vi "Lift PID Control.vi"(0 "Motor DevRefs IN":T15, 5 "Operator Gamepad":T4, 7 "Lift Potentionmeter":T1, 9 "Lift Deadband":dbl, 11 "Gains":cluster{"P":dbl, "I":dbl, "D":dbl}, 12 "Time to Wait":i32, 13 "Limit":dbl) -> (4 "Motor DevRefs OUT":T15, 10 "Tolerable?":bool)   [LabVIEW 2014]
uses:
  <vilib>/Rock Robotics/WPI/MotorControl/WPI_MotorControlDeviceRef.ctl
  <vilib>/Rock Robotics/WPI/MotorControl/WPI_MotorControlType.ctl
  <vilib>/Rock Robotics/SystemInterfaces/Typedef/FPGA_TypedefDigitalModule.ctl
  <vilib>/Rock Robotics/SystemInterfaces/DIO/FPGA_DIOPWMChannel.ctl
  <vilib>/Rock Robotics/WPI/PWM/WPI_PWMDeadband.ctl
  <vilib>/Rock Robotics/WPI/CAN/Jaguar/SubVIs/WPI_CANJaguar_ControlMode.ctl
  <vilib>/Rock Robotics/WPI/CAN/TalonSRX/WPI_CANTalonSRX_APIControlMode.ctl
  <vilib>/Rock Robotics/WPI/PWM/WPI_PWMTransform_ConPane.ctl
  <vilib>/Rock Robotics/WPI/Joystick/WPI_JoystickDevRef.ctl
  <vilib>/Rock Robotics/WPI/Joystick/WPI_JoystickDeviceEnum.ctl
  <vilib>/Rock Robotics/WPI/Potentiometer/WPI_PotentiometerDevRef.ctl
  <vilib>/Rock Robotics/SystemInterfaces/Typedef/FPGA_TypedefAnalogModule.ctl
  <vilib>/Rock Robotics/SystemInterfaces/AI/FPGA_AIChannel.ctl
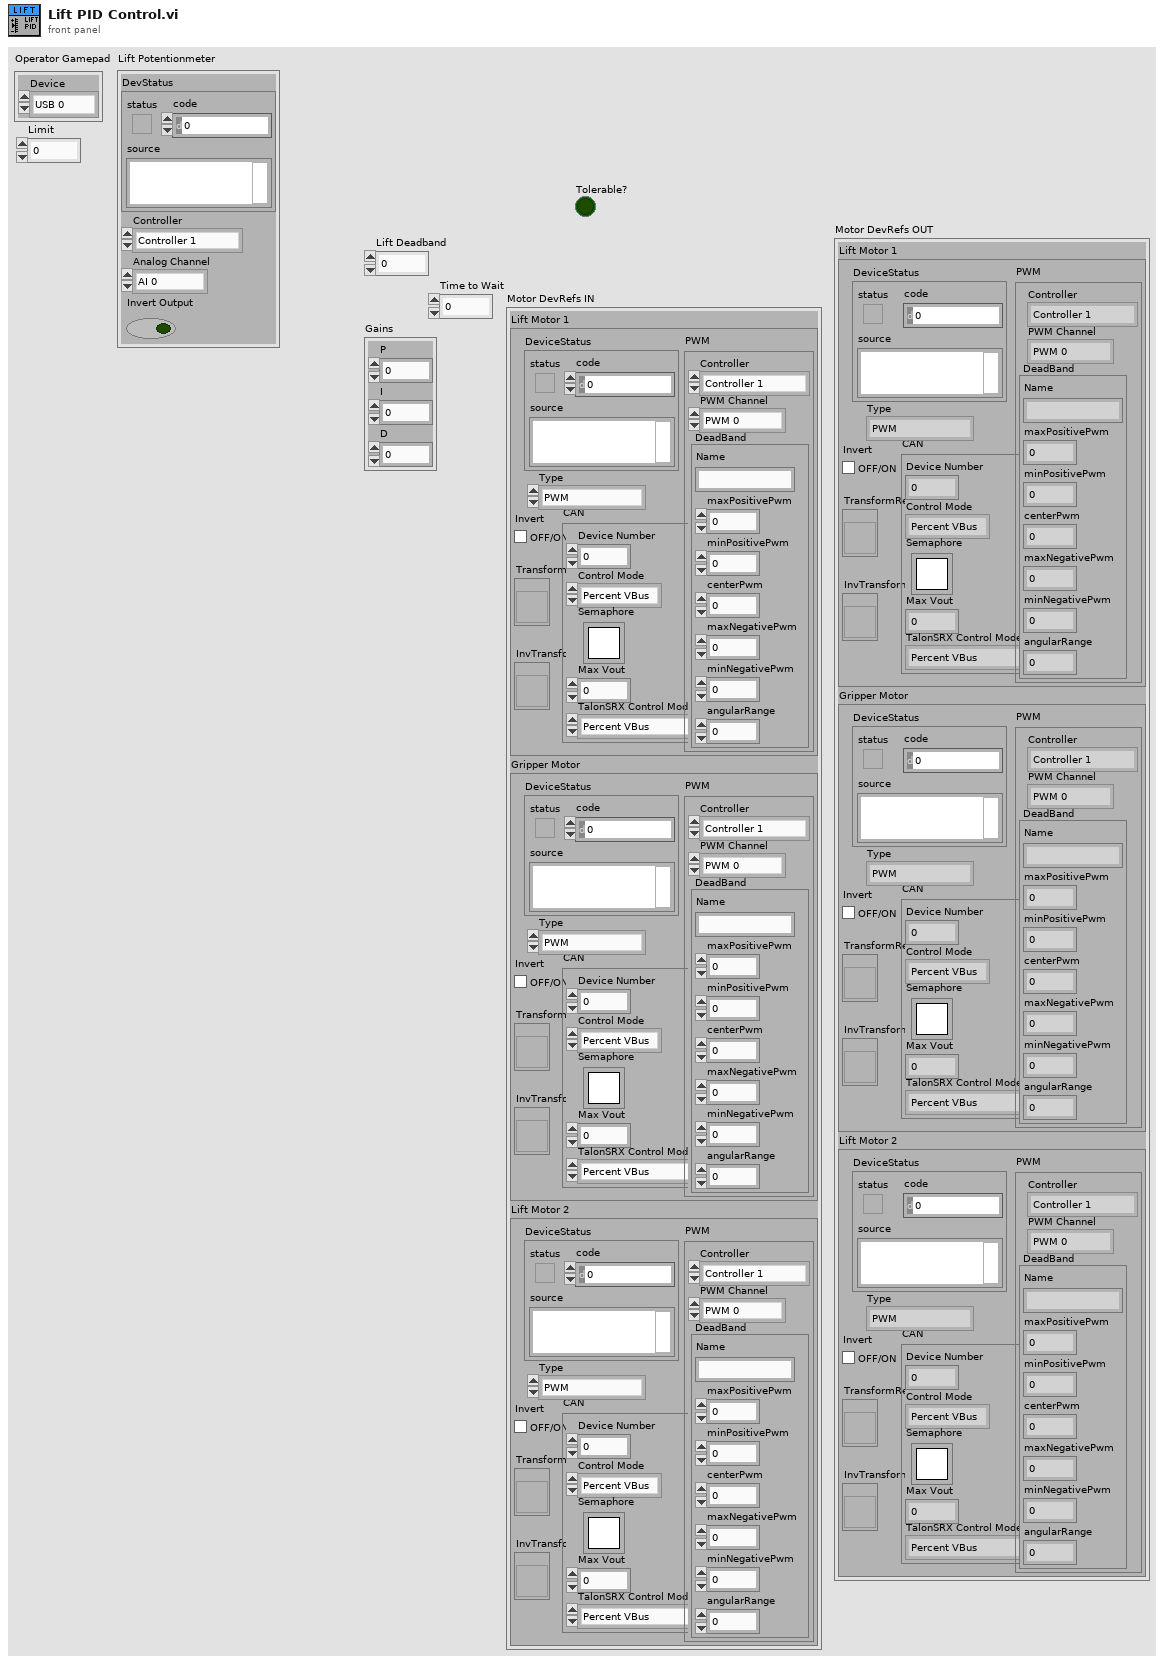
[diagram p1: front panel]
types:
  T1 = typedef "WPI_PotentiometerDevRef.ctl" = cluster{"DevStatus":errorcluster, "Controller":T2, "Analog Channel":T3, "Invert Output":bool}
  T2 = typedef "FPGA_TypedefAnalogModule.ctl" = enum16{"Controller 1"}
  T3 = typedef "FPGA_AIChannel.ctl" = enum8{"AI 0", "AI 1", "AI 2", "AI 3", "AI MXP 0", "AI MXP 1", "AI MXP 2", "AI MXP 3", "Invalid"}
  T4 = typedef "WPI_JoystickDevRef.ctl" = cluster{"Device":T5}
  T5 = typedef "WPI_JoystickDeviceEnum.ctl" = enum16{"USB 0", "USB 1", "USB 2", "USB 3", "USB 4", "USB 5"}
  T6 = typedef "WPI_MotorControlDeviceRef.ctl" = cluster{"DeviceStatus":errorcluster, "Type":T7, "PWM":cluster{"Controller":T8, "PWM Channel":T9, "DeadBand":T10}, "CAN":cluster{"Device Number":u8, "Control Mode":T11, "Semaphore":T12, "Max Vout":dbl, "TalonSRX Control Mode":T13}, "Invert":bool, "TransformRef":T14, "InvTransformRef":T14}
  T7 = typedef "WPI_MotorControlType.ctl" = enum16{"PWM", "CAN", "CANTalonSRX"}
  T8 = typedef "FPGA_TypedefDigitalModule.ctl" = enum16{"Controller 1"}
  T9 = typedef "FPGA_DIOPWMChannel.ctl" = enum8{"PWM 0", "PWM 1", "PWM 2", "PWM 3", "PWM 4", "PWM 5", "PWM 6", "PWM 7", "PWM 8", "PWM 9", "PWM MXP 0", "PWM MXP 1", "PWM MXP 2", "PWM MXP 3", "PWM MXP 4", "PWM MXP 5", "PWM MXP 6", "PWM MXP 7", "PWM MXP 8", "PWM MXP 9", "Invalid"}
  T10 = typedef "WPI_PWMDeadband.ctl" = cluster{"Name":string, "maxPositivePwm":i32, "minPositivePwm":i32, "centerPwm":i32, "maxNegativePwm":i32, "minNegativePwm":i32, "angularRange":u16}
  T11 = typedef "WPI_CANJaguar_ControlMode.ctl" = enum8{"Percent VBus", "Current", "Speed", "Position", "Voltage"}
  T12 = typedef "Semaphore RefNum" = refnum<k1>
  T13 = typedef "WPI_CANTalonSRX_APIControlMode.ctl" = enum8{"Percent VBus", "Speed", "Position", "Slave", "Unchanged / Invalid"}
  T14 = typedef "WPI_PWMTransform_ConPane.ctl" = refnum<vi>
  T15 = cluster{"Lift Motor 1":T6, "Gripper Motor":T6, "Lift Motor 2":T6}
  T16 = cluster{"Error":dbl, "millisecond timer value":u32, "To Shift Register":dbl}
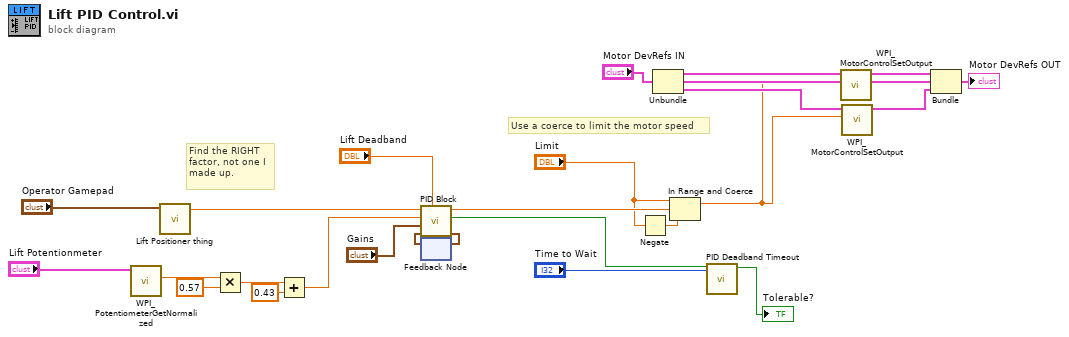
[diagram p0: block diagram]
diagram:
  # "Find the RIGHT\nfactor, not one I\nmade up."
  # "Use a coerce to limit the motor speed"
  n1 = call <vilib>:"WPI_PotentiometerGetNormalized.vi"("PotDevRef"="Lift Potentionmeter") -> ("Normalized Value"=w4:dbl)  [unwired: 8 in, 2 out]
  n2 = call "Lift Positioner thing.vi"("Operator Gamepad"="Operator Gamepad") -> ("Setpoint"=w6:dbl)  [unwired: 10 in]
  n3 = Multiply(x=w4, y=0.57) -> (x*y=w5:dbl)
  n4 = Add(x=w5, y=0.43) -> (x+y=w3:dbl)
  n5 = feedback #1() -> (w22:T16)  [unwired: 1 in]
  n6 = call "PID Block.vi"("Deadband"="Lift Deadband", "From Shift"=w22, "Gains"="Gains", "Position"=w3, "Setpoint"=w6) -> ("To Shift"=w23:T16, "Tolerable?"=w21:bool, "Output"=w10:dbl)  [unwired: 4 in]
  n7 = feedback-in #1(w23) -> ()
  n8 = Negate(x="Limit") -> (-x=w8:dbl)
  n9 = Unbundle("Motor DevRefs IN") -> ("Lift Motor 1"=w18:T6, "Lift Motor 2"=w17:T6)  [unwired: 1 out]
  n10 = In Range and Coerce(upper limit="Limit", x=w10, lower limit=w8) -> (coerced(x)=w9:dbl)  [unwired: 1 out]
  n11 = call "PID Deadband Timeout.vi"("Time to Wait"="Time to Wait", "In deadband range?"=w21) -> ("Deadband Timed-out"=→"Tolerable?":bool)  [unwired: 9 in]
  n12 = call <vilib>:"WPI_MotorControlSetOutput.vi"("Output"=w9, "MotorControlDevRef"=w18) -> ("MotorControlDevRef"=w15:T6)  [unwired: 7 in, 2 out]
  n13 = call <vilib>:"WPI_MotorControlSetOutput.vi"("Output"=w9, "MotorControlDevRef"=w17) -> ("MotorControlDevRef"=w14:T6)  [unwired: 7 in, 2 out]
  n14 = Bundle(cluster="Motor DevRefs IN", "Lift Motor 1"=w15, "Lift Motor 2"=w14) -> ()  [unwired: 1 in, 1 out]
  "Motor DevRefs OUT" <- "Motor DevRefs IN"
